vi "test wire straight.vi"   [LabVIEW 2017]
uses:
  <vilib>/Utility/miscctls.llb/LVRectTypeDef.ctl
  user.lib/_NEVSTOP/Communicable State Machine(CSM)/_csmHelper/CSM-Helper.lvclass/CSM-Helper.ctl
  user.lib/_NEVSTOP/Communicable State Machine(CSM)/_csmHelper/Properties/Read VI Ref.vi
  user.lib/_NEVSTOP/Communicable State Machine(CSM)/_csmHelper/API/Destroy.vi
  user.lib/_NEVSTOP/Communicable State Machine(CSM)/_csmHelper/API/Stop Undo.vi
  user.lib/_NEVSTOP/Communicable State Machine(CSM)/_csmHelper/API/Start Undo.vi
  user.lib/_NEVSTOP/Communicable State Machine(CSM)/_csmHelper/API/Open Block Diagram.vi
  user.lib/_NEVSTOP/Communicable State Machine(CSM)/_csmHelper/API/Create From VI Reference.vi
  user.lib/_NEVSTOP/Communicable State Machine(CSM)/_csmHelper/CSM-Helper.lvclass
  user.lib/_NEVSTOP/Communicable State Machine(CSM)/_csmHelper/Utility/_Support/Wire.llb/csmHelper-Wire.lvlib
  user.lib/_NEVSTOP/Communicable State Machine(CSM)/_csmHelper/Properties/Read Front Tunnel Internal TermRefs.vi
  user.lib/_NEVSTOP/Communicable State Machine(CSM)/_csmHelper/Properties/Read Case Structure Ref.vi
types:
  T1 = cluster{"Registration":refnum<vi>, "InternalData":refnum<vi>, "CSM Name":refnum<vi>, "Last Resp":refnum<vi>, "Remaining State":refnum<vi>, "Arguments":refnum<vi>, "Response Source":refnum<vi>, "Source CSM":refnum<vi>, "Selector":refnum<vi>, "Error":refnum<vi>}
  T2 = typedef "LVRectTypeDef.ctl" = cluster{"Left":i16, "Top":i16, "Right":i16, "Bottom":i16}
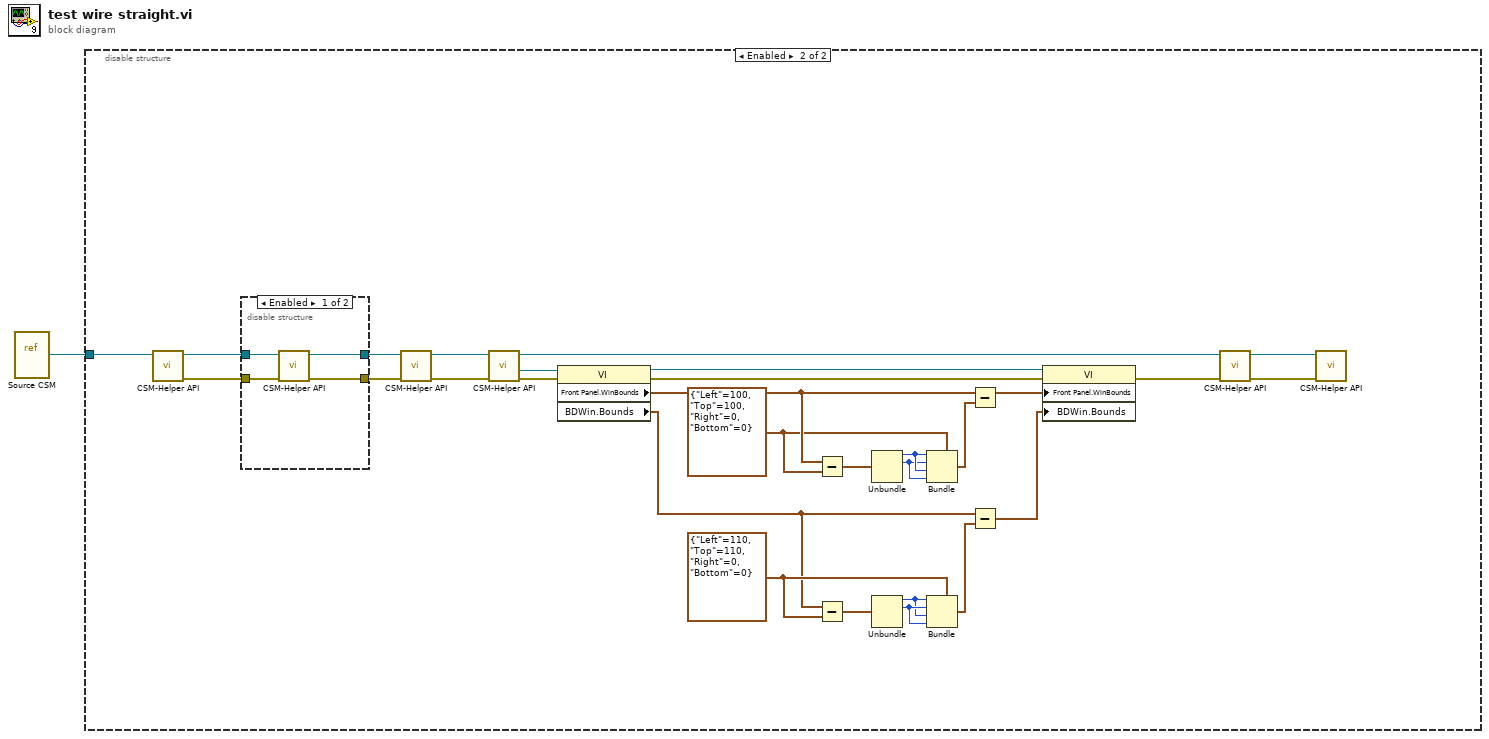
[diagram p0: block diagram]
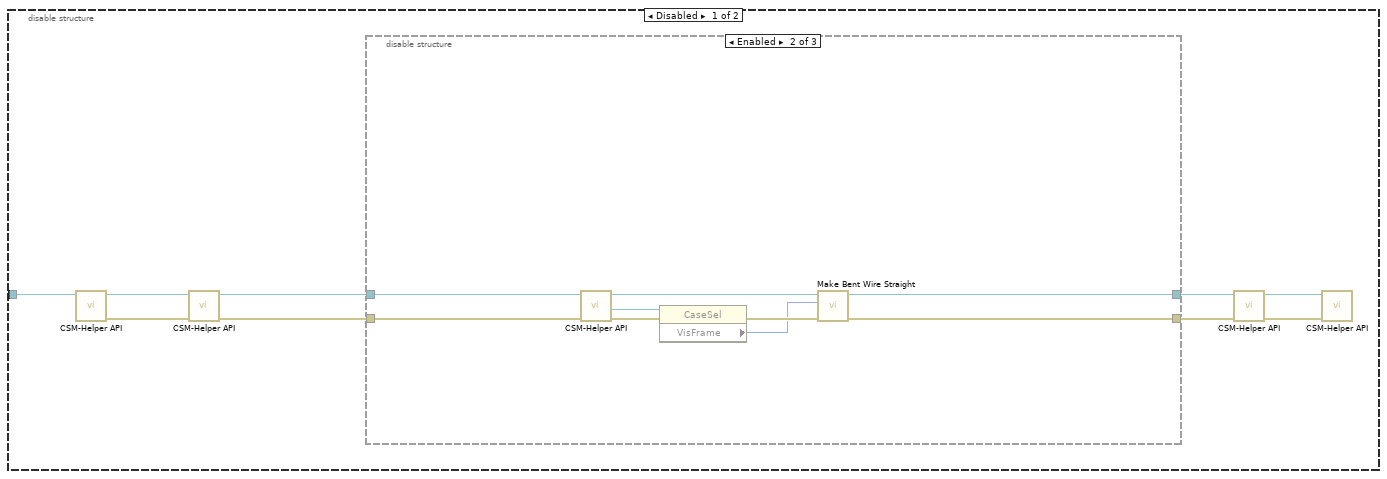
[diagram p2: hidden frame]
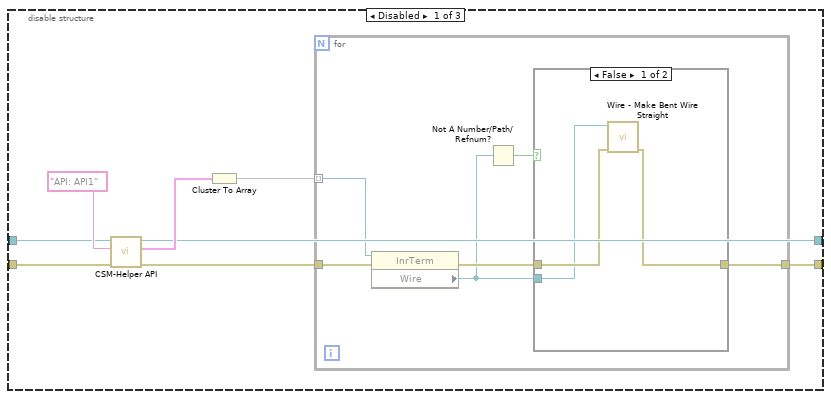
[diagram p3: hidden frame]
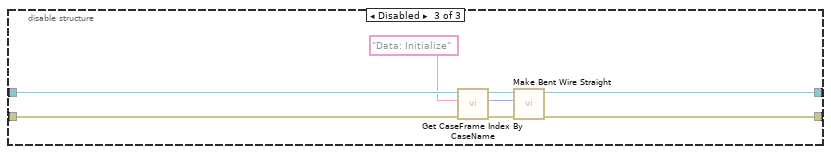
[diagram p5: hidden frame]
diagram:
  n1 = vi-ref "Source CSM.vi"() -> (w1:refnum<vi>)
  n2 = disable-structure shown="Enabled" {
    disable-tunnel: w1 -> [w10 w74]
    frame Disabled {
      n3 = call-poly "CSM-Helper API.vi"("VI"=w10) -> ("error out"=w8:errorcluster, "CSM-Helper.lvclass"=w9:refnum<class "CSM-Helper.lvclass">)  [unwired: 9 in]
      n4 = call-poly "CSM-Helper API.vi"("error in (no error)"=w8, "CSM-Helper in"=w9) -> ("error out"=w3:errorcluster, "CSM-Helper out"=w4:refnum<class "CSM-Helper.lvclass">)  [unwired: 8 in]
      n5 = disable-structure shown="Enabled" {
        disable-tunnel: [w17 w37 w45] -> w5
        disable-tunnel: w4 -> [w14 w34 w43]
        disable-tunnel: w3 -> [w13 w35 w41]
        disable-tunnel: [w12 w36 w44] -> w2
        frame Disabled {
          n6 = call-poly "CSM-Helper API.vi"("error in (no error)"=w13, "case"="API: API1", "CSM-Helper in"=w14) -> ("error out"=w16:errorcluster, "Front Tunnels"=w18:T1, "CSM-Helper out"=w12:refnum<class "CSM-Helper.lvclass">)  [unwired: 6 in]
          n7 = Cluster To Array(cluster=w18) -> (array=w11:refnum<vi>[])
          n8 = for {
            tunnel: w11 -> [w21] mode=indexing
            tunnel: w16 -> [w23]
            tunnel: [w24] -> w17
            n9 = property class="InrTerm"(reference=w21, error in=w23) -> (error out=w22:errorcluster, "Wire"=w20:refnum<vi>)  [unwired: 1 out]
            n10 = Not A Number/Path/Refnum?(number/path/refnum=w20) -> (NaN/Path/Refnum?=w19:bool)
            n11 = case shown="False" w19 {
              tunnel: [w27 w28] -> w24
              tunnel: w22 -> [w26 w28]
              tunnel: w20 -> [w25 _]
              frame False {
                n12 = call "Wire - Make Bent Wire Straight.vi"("error in (no error)"=w26, "Wire in"=w25) -> ("error out"=w27:errorcluster)  [unwired: 8 in, 1 out]
              }
              frame True {
              }
            }
          }
        }
        frame Enabled {
          n13 = call-poly "CSM-Helper API.vi"("error in (no error)"=w35, "CSM-Helper in"=w34) -> ("error out"=w33:errorcluster, "Case Structure"=w30:refnum<vi>, "CSM-Helper out"=w32:refnum<class "CSM-Helper.lvclass">)  [unwired: 7 in]
          n14 = property class="CaseSel"(reference=w30, error in=w33) -> (error out=w31:errorcluster, "VisFrame"=w29:u32)  [unwired: 1 out]
          n15 = call "Make Bent Wire Straight.vi"("error in (no error)"=w31, "Index (-1 For All)"=w29, "CSM-Helper In"=w32) -> ("error out"=w37:errorcluster, "CSM-Helper Out"=w36:refnum<class "CSM-Helper.lvclass">)  [unwired: 7 in]
        }
        frame Disabled {
          n16 = call "Get CaseFrame Index By CaseName.vi"("error in (no error)"=w41, "CASE"="Data: Initialize" ("case"), "CSM-Helper in"=w43) -> ("error out"=w42:errorcluster, "index"=w39:i32, "CSM-Helper out"=w40:refnum<class "CSM-Helper.lvclass">)  [unwired: 5 in, 1 out]
          n17 = call "Make Bent Wire Straight.vi"("error in (no error)"=w42, "Index (-1 For All)"=w39, "CSM-Helper In"=w40) -> ("error out"=w45:errorcluster, "CSM-Helper Out"=w44:refnum<class "CSM-Helper.lvclass">)  [unwired: 7 in]
        }
      }
      n18 = call-poly "CSM-Helper API.vi"("error in (no error)"=w5, "CSM-Helper in"=w2) -> ("error out"=w6:errorcluster, "CSM-Helper out"=w7:refnum<class "CSM-Helper.lvclass">)  [unwired: 8 in]
      n19 = call-poly "CSM-Helper API.vi"("error in (no error)"=w6, "CSM-Helper in"=w7) -> ()  [unwired: 8 in, 2 out]
    }
    frame Enabled {
      w49 = T2 {"Left"=110, "Top"=110, "Right"=0, "Bottom"=0} ("Front Panel Window:Window Bounds")
      w56 = T2 {"Left"=100, "Top"=100, "Right"=0, "Bottom"=0} ("Front Panel Window:Window Bounds")
      n20 = call-poly "CSM-Helper API.vi"("VI"=w74) -> ("error out"=w66:errorcluster, "CSM-Helper.lvclass"=w65:refnum<class "CSM-Helper.lvclass">)  [unwired: 9 in]
      n21 = disable-structure shown="Enabled" {
        disable-tunnel: w66 -> [w78 w79]
        disable-tunnel: w65 -> [w77 w80]
        disable-tunnel: [w76 w79] -> w64
        disable-tunnel: [w75 w80] -> w63
        frame Enabled {
          n22 = call-poly "CSM-Helper API.vi"("error in (no error)"=w78, "CSM-Helper in"=w77) -> ("error out"=w76:errorcluster, "CSM-Helper out"=w75:refnum<class "CSM-Helper.lvclass">)  [unwired: 8 in]
        }
        frame Disabled {
        }
      }
      n23 = call-poly "CSM-Helper API.vi"("error in (no error)"=w64, "CSM-Helper in"=w63) -> ("error out"=w71:errorcluster, "CSM-Helper out"=w70:refnum<class "CSM-Helper.lvclass">)  [unwired: 8 in]
      n24 = call-poly "CSM-Helper API.vi"("error in (no error)"=w71, "CSM-Helper in"=w70) -> ("error out"=w69:errorcluster, "VI"=w67:refnum<vi>, "CSM-Helper out"=w68:refnum<class "CSM-Helper.lvclass">)  [unwired: 7 in]
      n25 = property class="VI"(reference=w67, error in=w69) -> (reference out=w62:refnum<vi>, error out=w61:errorcluster, "Front Panel.WinBounds"=w58:T2, "BDWin.Bounds"=w47:T2)
      n26 = Subtract(x=w58, y=w56) -> (x-y=w57:T2)
      n27 = Subtract(x=w47, y=w49) -> (x-y=w48:T2)
      n28 = Unbundle(w57) -> ("Left"=w55:i16, "Top"=w54:i16)  [unwired: 2 out]
      n29 = Unbundle(w48) -> ("Left"=w50:i16, "Top"=w51:i16)  [unwired: 2 out]
      n30 = Bundle(cluster=w56, "Left"=w55, "Top"=w54, "Right"=w55, "Bottom"=w54) -> (w53:T2)
      n31 = Bundle(cluster=w49, "Left"=w50, "Top"=w51, "Right"=w50, "Bottom"=w51) -> (w52:T2)
      n32 = Subtract(x=w58, y=w53) -> (x-y=w59:T2)
      n33 = Subtract(x=w47, y=w52) -> (x-y=w46:T2)
      n34 = property class="VI"(reference=w62, error in=w61, "Front Panel.WinBounds"=w59, "BDWin.Bounds"=w46) -> (error out=w60:errorcluster)  [unwired: 1 out]
      n35 = call-poly "CSM-Helper API.vi"("error in (no error)"=w60, "CSM-Helper in"=w68) -> ("error out"=w72:errorcluster, "CSM-Helper out"=w73:refnum<class "CSM-Helper.lvclass">)  [unwired: 8 in]
      n36 = call-poly "CSM-Helper API.vi"("error in (no error)"=w72, "CSM-Helper in"=w73) -> ()  [unwired: 8 in, 2 out]
    }
  }
